vi "Teleop.vi"(10 "Match Info":T1={"Autonomous Elapsed Seconds"=0.0, "TeleOp Elapsed Seconds"=0.0, "Disabled Elapsed Seconds"=0.0, "Visited Autonomous"=FALSE, "Visited TeleOp"=FALSE, "Visited Disabled"=FALSE, "Autonomous Settings"={"Autonomous Style"=enum."Independent", "VI Refnum"=refnum}}, 11 "Call Context":T2) -> ()   [LabVIEW 2014]
doc: "This VI is called for each TeleOp packet received from the DS where the robot is not disabled. It is often used to read from the joysticks and update I/O or to update setpoints for timed control loops. It should complete and return within 20 milliseconds or it may miss DS packets."
uses:
  <vilib>/Rock Robotics/WPI/DriverStation/WPI_DriverStationDerivedRobotMode.ctl
  <vilib>/Rock Robotics/WPI/DriverStation/WPI_DriverStationMatch Info.ctl
  <vilib>/Rock Robotics/Network Tables/SD Read Number.vi
  <vilib>/Rock Robotics/WPI/RobotDrive/WPI_RobotDriveGetSetRefNum.vi
  <vilib>/Rock Robotics/WPI/Joystick/WPI_JoystickGetSetRefNum.vi
  <vilib>/Rock Robotics/Network Tables/SD Write Numeric Array.vi
  <vilib>/Rock Robotics/Network Tables/SD Write Boolean Array.vi
  <vilib>/Rock Robotics/WPI/RobotDrive/WPI_RobotDriveArcadeDrive_Standard(NoSaturation).vi
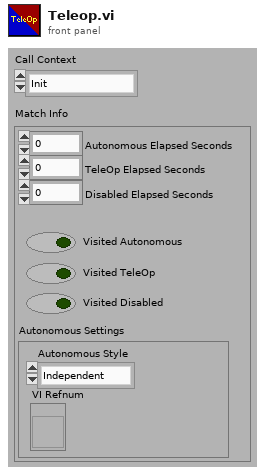
[diagram p1: front panel]
types:
  T1 = typedef "WPI_DriverStationMatch Info.ctl" = cluster{"Autonomous Elapsed Seconds":dbl, "TeleOp Elapsed Seconds":dbl, "Disabled Elapsed Seconds":dbl, "Visited Autonomous":bool, "Visited TeleOp":bool, "Visited Disabled":bool, "Autonomous Settings":cluster{"Autonomous Style":enum16{"Iterative", "Independent"}, "VI Refnum":refnum<vi>}}
  T2 = typedef "WPI_DriverStationDerivedRobotMode.ctl" = enum16{"Init", "Execute", "Stop"}
  T3 = typedef "WPI_RobotDriveDevRef.ctl" = cluster{"DevStatus":errorcluster, "Motors[]":T4[], "Square Inputs":bool, "Max Output":dbl}
  T4 = typedef "WPI_MotorControlDeviceRef.ctl" = cluster{"DeviceStatus":errorcluster, "Type":T5, "PWM":cluster{"Controller":T6, "PWM Channel":T7, "DeadBand":T8}, "CAN":cluster{"Device Number":u8, "Control Mode":T9, "Semaphore":T10, "Max Vout":dbl, "TalonSRX Control Mode":T11}, "Invert":bool, "TransformRef":T12, "InvTransformRef":T12}
  T5 = typedef "WPI_MotorControlType.ctl" = enum16{"PWM", "CAN", "CANTalonSRX"}
  T6 = typedef "FPGA_TypedefDigitalModule.ctl" = enum16{"Controller 1"}
  T7 = typedef "FPGA_DIOPWMChannel.ctl" = enum8{"PWM 0", "PWM 1", "PWM 2", "PWM 3", "PWM 4", "PWM 5", "PWM 6", "PWM 7", "PWM 8", "PWM 9", "PWM MXP 0", "PWM MXP 1", "PWM MXP 2", "PWM MXP 3", "PWM MXP 4", "PWM MXP 5", "PWM MXP 6", "PWM MXP 7", "PWM MXP 8", "PWM MXP 9", "Invalid"}
  T8 = typedef "WPI_PWMDeadband.ctl" = cluster{"Name":string, "maxPositivePwm":i32, "minPositivePwm":i32, "centerPwm":i32, "maxNegativePwm":i32, "minNegativePwm":i32, "angularRange":u16}
  T9 = typedef "WPI_CANJaguar_ControlMode.ctl" = enum8{"Percent VBus", "Current", "Speed", "Position", "Voltage"}
  T10 = typedef "Semaphore RefNum" = refnum<k1>
  T11 = typedef "WPI_CANTalonSRX_APIControlMode.ctl" = enum8{"Percent VBus", "Speed", "Position", "Slave", "Unchanged / Invalid"}
  T12 = typedef "WPI_PWMTransform_ConPane.ctl" = refnum<vi>
  T13 = typedef "WPI_JoystickDevRef.ctl" = cluster{"Device":T14}
  T14 = typedef "WPI_JoystickDeviceEnum.ctl" = enum16{"USB 0", "USB 1", "USB 2", "USB 3", "USB 4", "USB 5"}
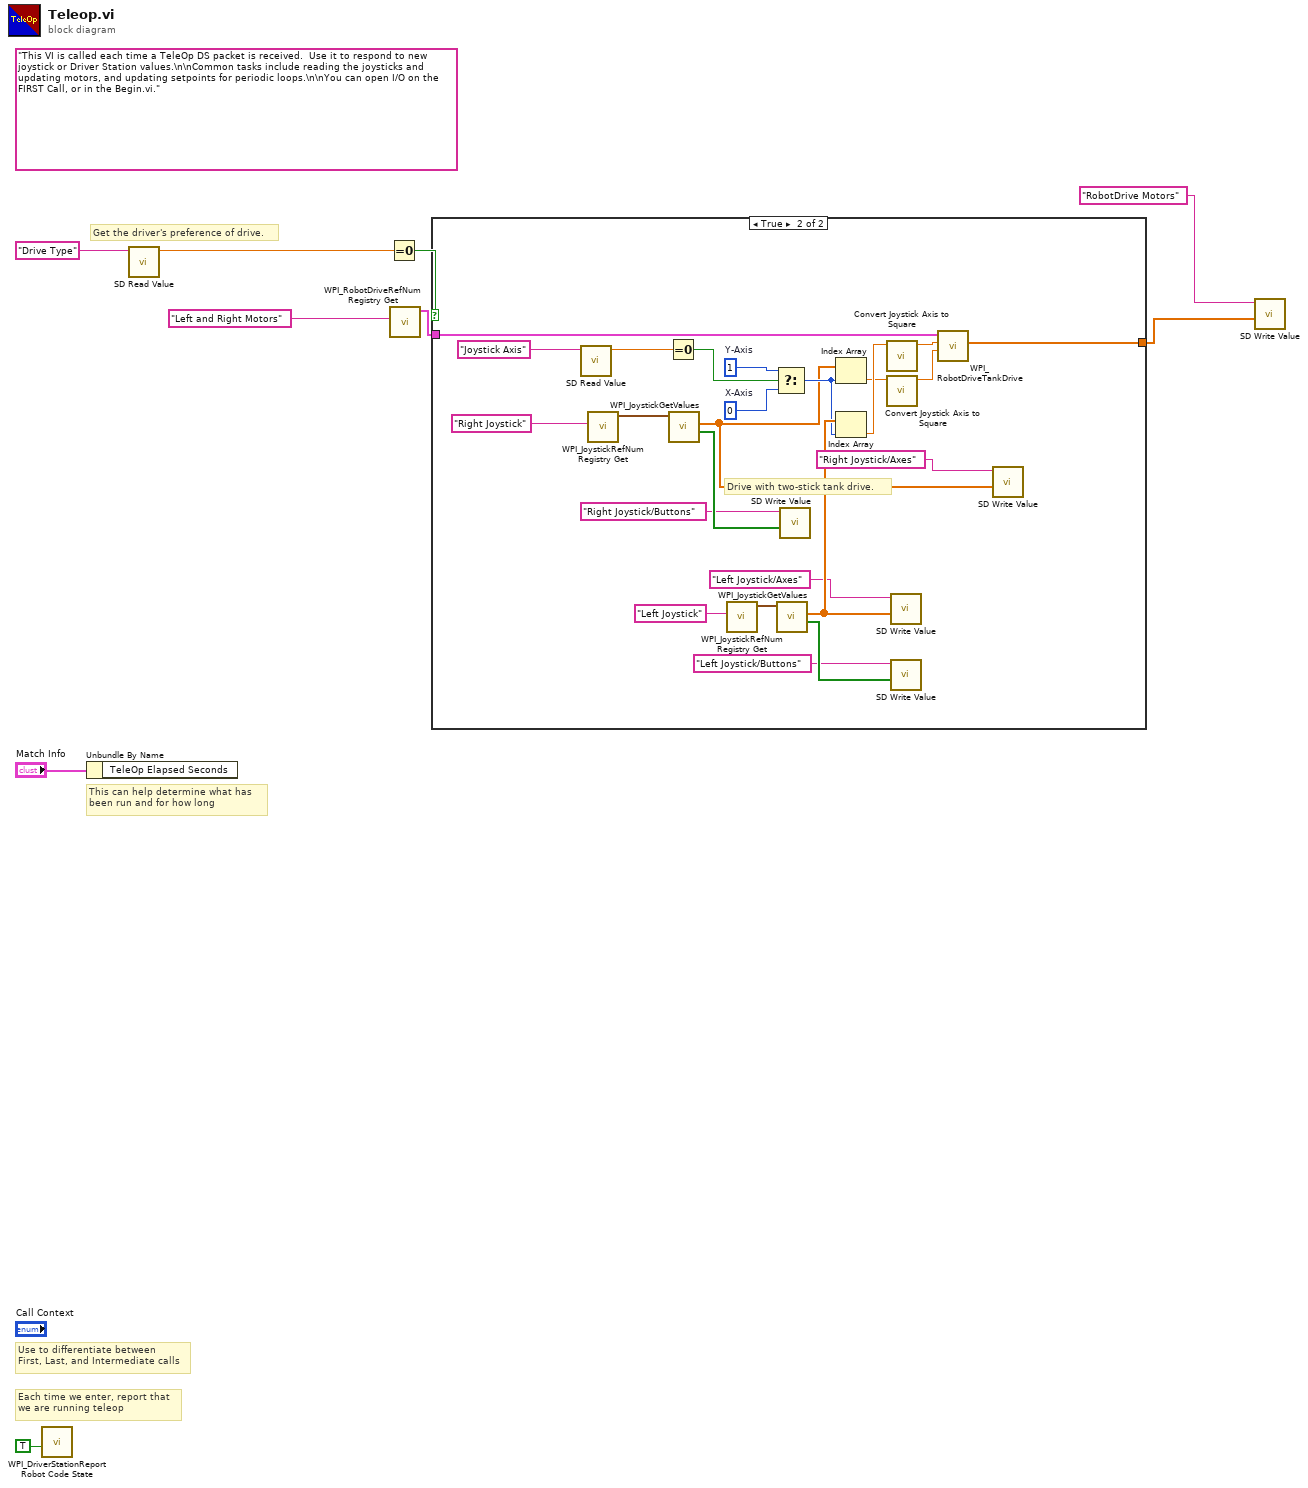
[diagram p0: block diagram]
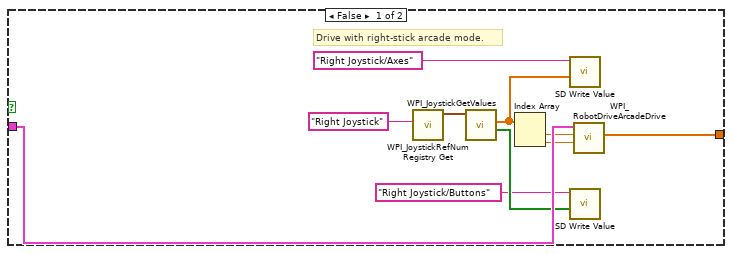
[diagram p2: hidden frame]
diagram:
  (unwired) "This VI is called each time a TeleOp DS packet is received.  Use it to respond to new joystick or Driver Station values.\n\nCommon tasks include reading the joysticks and updating motors, and updating setpoints for periodic loops.\n\nYou can open I/O on the FIRST Call, or in the Begin.vi."
  # "Get the driver's preference of drive."
  # "Each time we enter, report that\nwe are running teleop"
  # "Use to differentiate between\nFirst, Last, and Intermediate calls"
  # "This can help determine what has\nbeen run and for how long"
  n1 = call <vilib>:"WPI_DriverStationReport Robot Code State.vi"("TeleOp"=TRUE ("Autonomous")) -> ()  [unwired: 10 in, 1 out]
  n2 = Unbundle By Name("Match Info") -> ()  [unwired: 1 out]
  n3 = call-poly <vilib>:"SD Read Value.vi"("Name"="Drive Type") -> ("Numeric"=w1:dbl)  [unwired: 8 in, 2 out]
  n4 = Equal To 0?(x=w1) -> (x = 0?=w7:bool)
  n5 = call <vilib>:"WPI_RobotDriveRefNum Registry Get.vi"("refnum name"="Left and Right Motors") -> ("RobotDriveDevRef"=w3:T3)  [unwired: 1 in, 9 out]
  n6 = case shown="True" w7 {
    tunnel: [w18 w32] -> w4
    tunnel: w3 -> [w19 w31]
    frame False {
      # "Drive with right-stick arcade mode."
      n7 = call <vilib>:"WPI_JoystickRefNum Registry Get.vi"("refnum name"="Right Joystick") -> ("JoystickDevRef"=w10:T13)  [unwired: 1 in, 9 out]
      n8 = call <vilib>:"WPI_JoystickGetValues.vi"("JoystickDevRef"=w10) -> ("Buttons"=w16:bool[], "Axes"=w14:dbl[])  [unwired: 6 in, 3 out]
      n9 = Index Array(array=w14) -> (element #1=w13:dbl, element #2=w12:dbl)  [unwired: 2 in]
      n10 = call-poly <vilib>:"SD Write Value.vi"("Numeric Array"=w14, "Name"="Right Joystick/Axes") -> ()  [unwired: 8 in, 2 out]
      n11 = call-poly <vilib>:"SD Write Value.vi"("Boolean Array"=w16, "Name"="Right Joystick/Buttons") -> ()  [unwired: 8 in, 2 out]
      n12 = call-poly <vilib>:"WPI_RobotDriveArcadeDrive.vi"("Y axis value"=w12, "X axis value"=w13, "RobotDriveDevRef"=w19) -> ("Motor Values"=w18:dbl[])  [unwired: 6 in, 2 out]
    }
    frame True {
      w35 = 0  # X-Axis
      w36 = 1  # Y-Axis
      # "Drive with two-stick tank drive."
      n13 = call-poly <vilib>:"SD Read Value.vi"("Name"="Joystick Axis") -> ("Numeric"=w24:dbl)  [unwired: 8 in, 2 out]
      n14 = call <vilib>:"WPI_JoystickRefNum Registry Get.vi"("refnum name"="Right Joystick") -> ("JoystickDevRef"=w25:T13)  [unwired: 1 in, 9 out]
      n15 = Equal To 0?(x=w24) -> (x = 0?=w34:bool)
      n16 = call <vilib>:"WPI_JoystickGetValues.vi"("JoystickDevRef"=w25) -> ("Buttons"=w29:bool[], "Axes"=w27:dbl[])  [unwired: 6 in, 3 out]
      n17 = call <vilib>:"WPI_JoystickRefNum Registry Get.vi"("refnum name"="Left Joystick") -> ("JoystickDevRef"=w38:T13)  [unwired: 1 in, 9 out]
      n18 = Select(t=w36, s=w34, f=w35) -> (s? t:f=w33:i32)
      n19 = call <vilib>:"WPI_JoystickGetValues.vi"("JoystickDevRef"=w38) -> ("Buttons"=w42:bool[], "Axes"=w40:dbl[])  [unwired: 6 in, 3 out]
      n20 = call-poly <vilib>:"SD Write Value.vi"("Boolean Array"=w29, "Name"="Right Joystick/Buttons") -> ()  [unwired: 8 in, 2 out]
      n21 = Index Array(array=w27, index=w33) -> (element=w21:dbl)
      n22 = Index Array(array=w40, index=w33) -> (element=w23:dbl)
      n23 = call "Convert Joystick Axis to Square.vi"("Joystick Axis"=w23) -> ("Squared"=w22:dbl)  [unwired: 10 in]
      n24 = call "Convert Joystick Axis to Square.vi"("Joystick Axis"=w21) -> ("Squared"=w20:dbl)  [unwired: 10 in]
      n25 = call-poly <vilib>:"SD Write Value.vi"("Numeric Array"=w40, "Name"="Left Joystick/Axes") -> ()  [unwired: 8 in, 2 out]
      n26 = call-poly <vilib>:"SD Write Value.vi"("Boolean Array"=w42, "Name"="Left Joystick/Buttons") -> ()  [unwired: 8 in, 2 out]
      n27 = call <vilib>:"WPI_RobotDriveTankDrive.vi"("Right axis value"=w20, "Left axis value"=w22, "RobotDriveDevRef"=w31) -> ("Motor Values"=w32:dbl[])  [unwired: 6 in, 2 out]
      n28 = call-poly <vilib>:"SD Write Value.vi"("Numeric Array"=w27, "Name"="Right Joystick/Axes") -> ()  [unwired: 8 in, 2 out]
    }
  }
  n29 = call-poly <vilib>:"SD Write Value.vi"("Numeric Array"=w4, "Name"="RobotDrive Motors") -> ()  [unwired: 8 in, 2 out]
